vi "MPXsetSignalDC.vi"(1 "Waveform":u16(ring)=3 items=["Sine", "Rectangle", "SRS-Signal"], 2 "MPX COM-Port":refnum<visa-resource-name>="COM5") -> (0 "MPX COM-Port dup":refnum<visa-resource-name>="COM5")   [LabVIEW 2015]
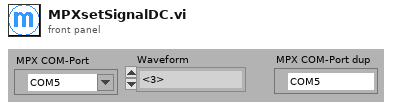
[diagram p1: front panel]
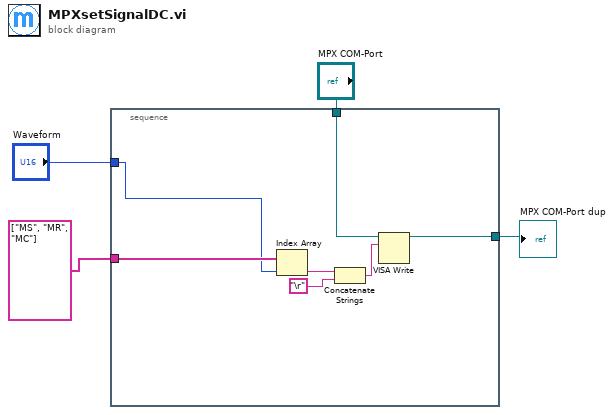
[diagram p0: block diagram]
diagram:
  n1 = stacked-sequence {
    tunnel: string[] ["MS", "MR", "MC"] -> [w11]
    tunnel: "MPX COM-Port" -> [w7]
    tunnel: "Waveform" -> [w6]
    tunnel: [w5] -> w1
    frame #0 {
      n2 = Index Array(array=w11, index=w6) -> (element=w10:string)
      n3 = Concatenate Strings(w10, "\r") -> (w8:string)
      n4 = VISA Write(VISA resource name=w7, write buffer=w8) -> (VISA resource name out=w5:refnum<visa-resource-name>)  [unwired: 1 in, 2 out]
    }
  }
  "MPX COM-Port dup" <- w1
